vi "Operation Event Enable Query.vi"(0 "VISA resource name":refnum<visa-resource-name>, 11 "error in (no error)":errorcluster) -> (4 "VISA resource name out":refnum<visa-resource-name>, 6 "Operation Event Enable":T1, 15 "error out":errorcluster)   [LabVIEW 2018, in "XP Power PLS600.lvlib"]
doc: "Queries the Operation Event Enable register. Returns the decimal value of binary-weighted sum of bits.\n\nThe Operation Event Enable register consists of the following 16 bits.\n\nBit 0: Calibrating\nBit 1: Setting\nBit 2: Ranging \nBit 3: Sweeping\nBit 4: Measuring\nBit 5: Waiting for Trigger \nBit 6: Waiting for Arm\nBit 7: Correcting\nBit 8: Output Enabled\nBit 9: Constant Voltage\nBit 10: Constant Current\nBit 11: Reserved\nBit 12: Reserved\nBit 13: Instrument Summary\nBit 14: Program Running\nBit 15: Reserved"
uses:
  XP Power PLS600.lvlib
panel:
  # "Bit 0:  Calibrating\nBit 1:  Setting\nBit 2:  Ranging\t\nBit 3:  Sweeping\nBit 4:\t\tMeasuring\nBit 5:  Waiting for Trigger\t\nBit 6:  Waiting for Arm\nBit 7:  Correcting\nBit 8:  Output Enabled\nBit 9:  Constant Voltage\nBit 10:  Constant Current\nBit 11:  Reserved\nBit 12:  Reserved\nBit 13:  Instrument Summary\nBit 14:  Program Running\nBit 15:  Reserved"
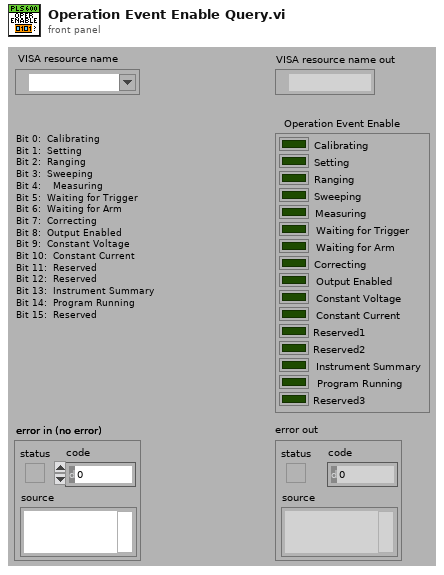
[diagram p1: front panel]
types:
  T1 = cluster{"Calibrating":bool, "Setting":bool, "Ranging":bool, "Sweeping":bool, "Measuring":bool, "Waiting for Trigger":bool, "Waiting for Arm":bool, "Correcting":bool, "Output Enabled":bool, "Constant Voltage":bool, "Constant Current":bool, "Reserved1":bool, "Reserved2":bool, "Instrument Summary":bool, "Program Running":bool, "Reserved3":bool}
  T2 = cluster{"Boolean array[0]":bool, "Boolean array[1]":bool, "Boolean array[2]":bool, "Boolean array[3]":bool, "Boolean array[4]":bool, "Boolean array[5]":bool, "Boolean array[6]":bool, "Boolean array[7]":bool, "Boolean array[8]":bool, "Boolean array[9]":bool, "Boolean array[10]":bool, "Boolean array[11]":bool, "Boolean array[12]":bool, "Boolean array[13]":bool, "Boolean array[14]":bool, "Boolean array[15]":bool}
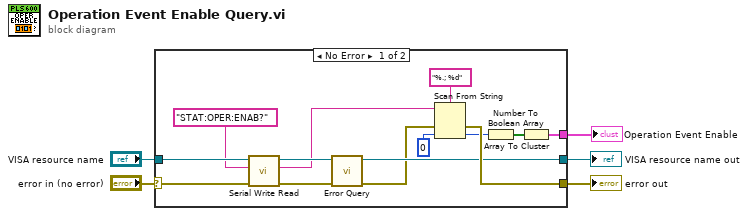
[diagram p0: block diagram]
diagram:
  n1 = case shown="No Error" "error in (no error)" {
    selector: "error in (no error)" -> [w10 w21]
    tunnel: [w16 _] -> w1
    tunnel: "VISA resource name" -> [w11 w20]
    tunnel: [w8 w20] -> w4
    tunnel: [w15 w21] -> w3
    frame No Error {
      n2 = call "Serial Write Read.vi"("error in (no error)"=w10, "Write Buffer"="STAT:OPER:ENAB?" ("Command to Send (empty)"), "VISA resource name"=w11) -> ("error out"=w13:errorcluster, "Read Buffer"=w6:string, "VISA resource name out"=w12:refnum<visa-resource-name>)  [unwired: 6 in]
      n3 = call "Error Query.vi"("error in (no error)"=w13, "VISA resource name"=w12) -> ("error out"=w7:errorcluster, "VISA resource name out"=w8:refnum<visa-resource-name>)  [unwired: 6 in, 2 out]
      n4 = Scan From String(format string="%.; %d" ("Format String"), input string=w6, error in=w7, default 1=u16 0 ("default value 1")) -> (error out=w15:errorcluster, output 1=w14:u16)  [unwired: 1 in, 2 out]
      n5 = Number To Boolean Array(number=w14) -> (Boolean array=w17:bool[])
      n6 = Array To Cluster(array=w17) -> (cluster=w16:T2)
    }
    frame Error {
    }
  }
  "error out" <- w3
  "VISA resource name out" <- w4
  "Operation Event Enable" <- w1
